vi "Pitot-static_to_Velocity.vi"(0 "Pressure Trans voltage":dbl[](array[numeric]) format="%.2f", 1 "Stat gauge Press mmH2O  (0)":dbl format="%.1f", 2 "Atmos Press mbar  (1000)":dbl=1000.0 format="%.1f", 3 "Temp  C  (20)":dbl=20.0 format="%.1f", 4 "Pressure Trans Calib const":dbl[](array[numeric]) format="%.6f") -> (5 "Velocity (m/s)":dbl[](array[numeric]) format="%.2f", 7 "Density Kg/m3":dbl format="%.2f")   [LabVIEW 2010]
doc: "this vi calculates the fluid velocity from the dynamic pressure measured with a pitot tube. Given a voltage array from the micro manometer and its calibration constants, it calculates the dynamic pressure, and knowing the temperature and absolute pressure of the fluid, calculates its velocity."
uses:
  Controls/Pressure_Units.ctl
panel:
  # "A              B"
  # "Instrument by PH. 18/2/94"
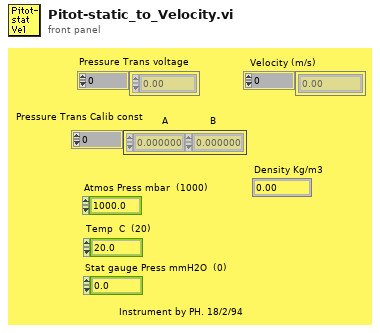
[diagram p1: front panel]
types:
  T1 = typedef "Pressure_Units.ctl" = enum16{"mmH2O", "mmHg", "Pa (N/m^2)", "mbar", "bar"}
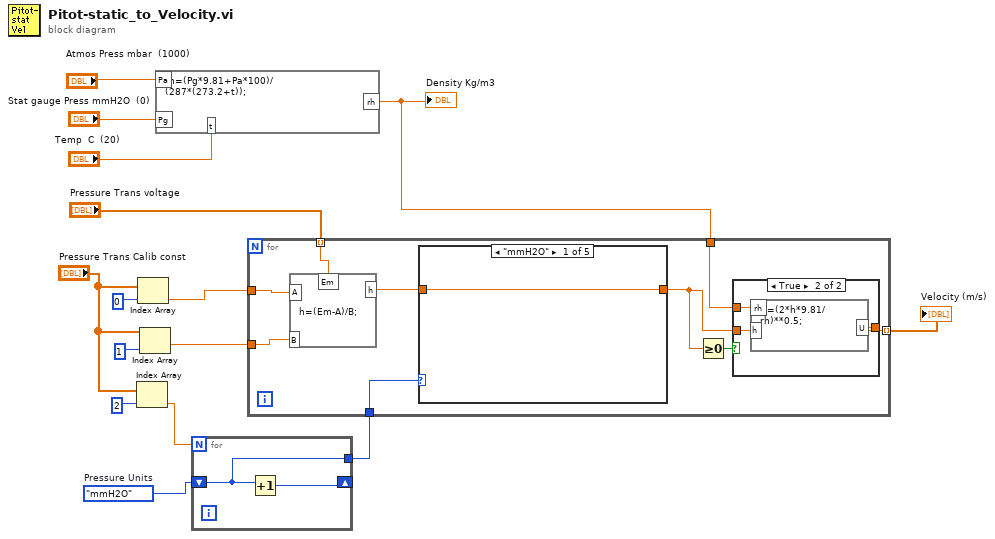
[diagram p0: block diagram]
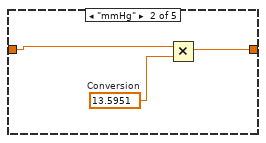
[diagram p2: hidden frame]
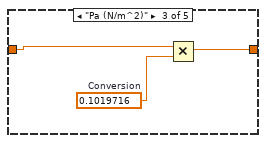
[diagram p3: hidden frame]
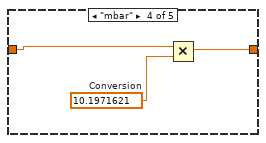
[diagram p4: hidden frame]
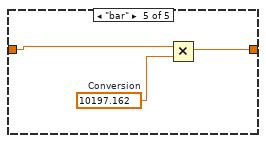
[diagram p5: hidden frame]
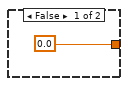
[diagram p6: hidden frame]
diagram:
  w3 = Pressure_Units."mmH2O"  # Pressure Units
  n1 = Index Array(array="Pressure Trans Calib const", index=2) -> (element=w2:dbl)
  n2 = Index Array(array="Pressure Trans Calib const", index=0) -> (element=w7:dbl)
  n3 = Index Array(array="Pressure Trans Calib const", index=1) -> (element=w6:dbl)
  n4 = formula code="rh=(Pg*9.81+Pa*100)/\n(287*(273.2+t));"("t"="Temp  C  (20)", "Pg"="Stat gauge Press mmH2O  (0)", "Pa"="Atmos Press mbar  (1000)") -> ("rh"=w11:dbl)
  "Density Kg/m3" <- w11
  n5 = for {
    N: w2 -> [_]
    shift-right: [w17] -> _
    shift-left: w3 -> [w16]
    tunnel: [w16] -> w1
    n6 = Increment(x=w16) -> (x+1=w17:T1)
  }
  n7 = for {
    tunnel: [w22] -> w10 mode=indexing
    tunnel: w11 -> [w23]
    tunnel: "Pressure Trans voltage" -> [w24] mode=indexing
    tunnel: w6 -> [w25]
    tunnel: w7 -> [w26]
    tunnel: w1 -> [w20]
    n8 = formula code="h=(Em-A)/B;"("Em"=w24, "B"=w25, "A"=w26) -> ("h"=w19:dbl)
    n9 = case shown="\"mmH2O\"" w20 {
      tunnel: [w27 w29 w32 w35 w38] -> w18
      tunnel: w19 -> [w27 w30 w33 w36 w39]
      frame "mmH2O" {
      }
      frame "mmHg" {
        w28 = 13.5951  # Conversion
        n10 = Multiply(x=w30, y=w28) -> (x*y=w29:dbl)
      }
      frame "Pa (N/m^2)" {
        w31 = 0.1019716  # Conversion
        n11 = Multiply(x=w33, y=w31) -> (x*y=w32:dbl)
      }
      frame "mbar" {
        w34 = 10.1971621  # Conversion
        n12 = Multiply(x=w36, y=w34) -> (x*y=w35:dbl)
      }
      frame "bar" {
        w37 = 10197.162  # Conversion
        n13 = Multiply(x=w39, y=w37) -> (x*y=w38:dbl)
      }
    }
    n14 = Greater Or Equal To 0?(x=w18) -> (x >= 0?=w21:bool)
    n15 = case shown="True" w21 {
      tunnel: w23 -> [_ w43]
      tunnel: [0.0 w42] -> w22
      tunnel: w18 -> [_ w41]
      frame False {
      }
      frame True {
        n16 = formula code="U=(2*h*9.81/rh)**0.5;"("rh"=w43, "h"=w41) -> ("U"=w42:dbl)
      }
    }
  }
  "Velocity (m/s)" <- w10
